vi "LabVLC - TerminateControl.vi"(2 "error in (no error)":errorcluster, 3 "LabVLC":T1={"media_ptr"=0, "vlc_inst_ptr"=0, "path in"=path "C:/Program Files (x86)/VideoLAN/VLC/libvlc.dll"}) -> (0 "error out":errorcluster)   [LabVIEW 2014]
doc: "Terminate the LabVLC player identified by the LabVLC cluster. Releases the VLC player library back to the OS. It is necessary to terminate LabVLC when you are completely finished with your VI, or when you want to change your video."
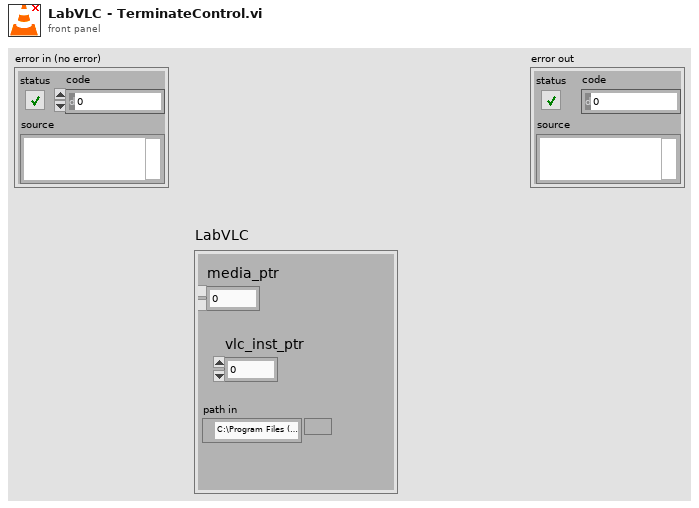
[diagram p1: front panel]
types:
  T1 = cluster{"media_ptr":i32, "vlc_inst_ptr":i32, "path in":path}
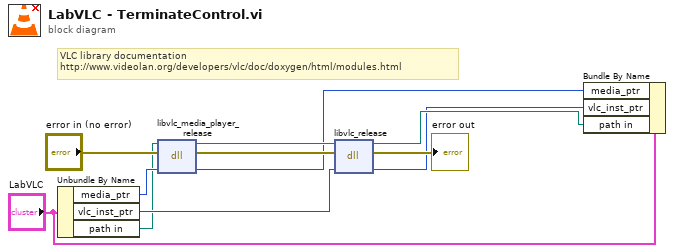
[diagram p0: block diagram]
diagram:
  # "VLC library documentation\nhttp://www.videolan.org/developers/vlc/doc/doxygen/html/modules.html"
  n1 = Unbundle By Name("LabVLC") -> ("media_ptr"=w2:i32, "vlc_inst_ptr"=w3:i32, "path in"=w1:path)
  n2 = dll-call lib="C:/Program Files (x86)/VideoLAN/VLC/libvlc.dll" fn="libvlc_media_player_release"(path in=w1, error in="error in (no error)", "media_pointer"=w2) -> (path out=w8:path, error out=w11:errorcluster, "media_pointer"=w4:i32)  [unwired: 2 in]
  n3 = dll-call lib="C:/Program Files (x86)/VideoLAN/VLC/libvlc.dll" fn="libvlc_release"(path in=w8, error in=w11, "vlc_inst_pointer"=w3) -> (path out=w6:path, error out=→"error out":errorcluster, "vlc_inst_pointer"=w5:i32)  [unwired: 2 in]
  n4 = Bundle By Name(cluster="LabVLC", "media_ptr"=w4, "vlc_inst_ptr"=w5, "path in"=w6) -> ()  [unwired: 1 out]
